vi "Check Wired Terminal.vi"(10 "Type Descriptor":T4, 11 "Terminal Type":variant) -> (3 "Terminal Status":T1)   [LabVIEW 2022 SP3, in "FlexBlocks Support.lvlib"]
uses:
  FlexBlocks Support.lvlib
  Type Descriptor.ctl
  Terminal Direction.ctl
  Value Mode.ctl
  Special Terminal.ctl
  Terminal Status.ctl
  Terminal State.ctl
  Terminal Draw Style.ctl
  <vilib>/Utility/Data Type/NI_Data Type.lvlib
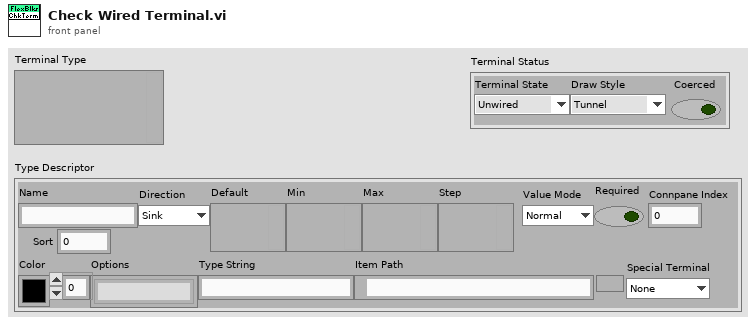
[diagram p1: front panel]
types:
  T1 = typedef "FlexBlocks Support.lvlib/Terminal Status.ctl" = cluster{"Terminal State":T2, "Draw Style":T3, "Coerced":bool}
  T2 = typedef "FlexBlocks Support.lvlib/Terminal State.ctl" = enum16{"Unwired", "BadType", "BadRef", "Channel", "Value", "Control Ref"}
  T3 = typedef "FlexBlocks Support.lvlib/Terminal Draw Style.ctl" = enum16{"Tunnel", "BadType", "BadRef", "Channel", "Value", "Control Ref"}
  T4 = typedef "FlexBlocks Support.lvlib/Type Descriptor.ctl" = cluster{"Name":string, "Direction":T5, "Default":variant, "Min":variant, "Max":variant, "Step":variant, "Value Mode":T6, "Color":u32, "Options":string[], "Type String":string, "Item Path":path, "Required":bool, "Connpane Index":i32, "Special Terminal":T7, "Sort":i32}
  T5 = typedef "FlexBlocks Support.lvlib/Terminal Direction.ctl" = enum16{"Sink", "Source"}
  T6 = typedef "FlexBlocks Support.lvlib/Value Mode.ctl" = enum16{"Normal", "Range", "Select"}
  T7 = typedef "FlexBlocks Support.lvlib/Special Terminal.ctl" = enum16{"None", "Action", "Init", "Tag", "State in", "State out", "Error"}
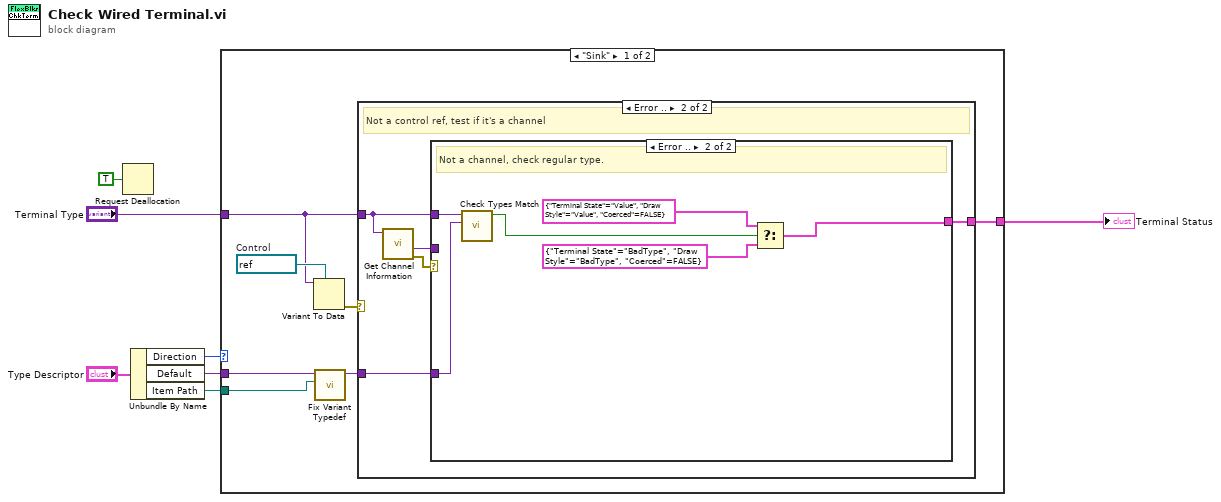
[diagram p0: block diagram]
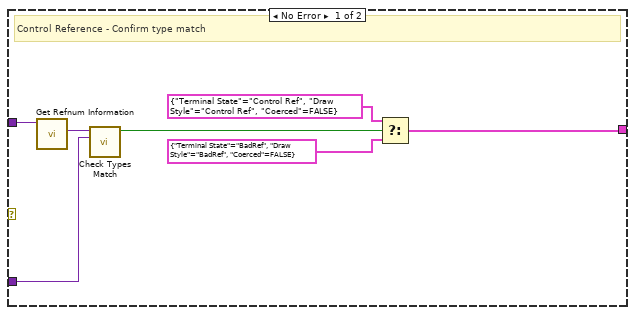
[diagram p2: hidden frame]
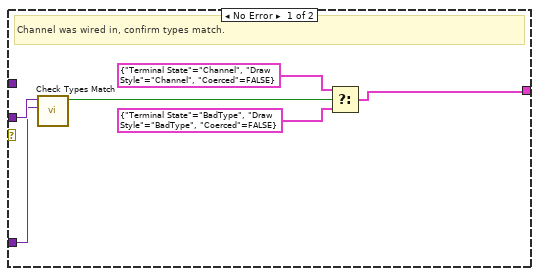
[diagram p3: hidden frame]
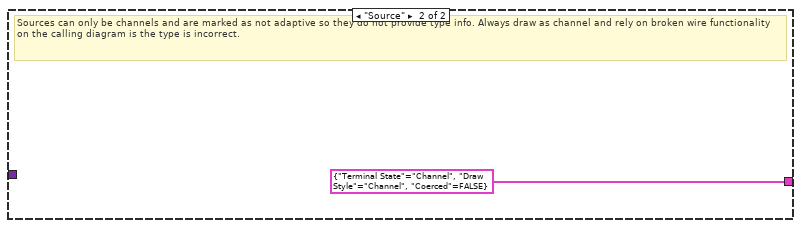
[diagram p4: hidden frame]
diagram:
  n1 = Request Deallocation(TRUE ("flag")) -> ()
  n2 = Unbundle By Name("Type Descriptor") -> ("Direction"=w1:T5, "Default"=w4:variant, "Item Path"=w3:path)
  n3 = case shown="\"Sink\"" w1 {
    tunnel: "Terminal Type" -> [w13 _]
    tunnel: w4 -> [w11 _]
    tunnel: w3 -> [w10 _]
    tunnel: [w8 T1 {"Terminal State"=enum."Channel", "Draw Style"=enum."Channel", "Coerced"=FALSE} ("Terminal Status")] -> w2
    frame "Sink" {
      w14 = refnum<vi> refnum  # Control
      n4 = Variant To Data(type=w14, Variant=w13) -> (error out=w12:errorcluster)  [unwired: 1 in, 1 out]
      n5 = call "Fix Variant Typedef.vi"("Item Path"=w10, "Default"=w11) -> ("Fixed Variant"=w9:variant)  [unwired: 9 in]
      n6 = case shown="Error .." w12 {
        tunnel: w13 -> [w21 w22]
        tunnel: w9 -> [w19 w24]
        tunnel: [w15 w23] -> w8
        frame No Error {
          # "Control Reference - Confirm type match"
          n7 = call <vilib>:"Get Refnum Information.vi"("variant"=w21) -> ("strict type"=w20:variant)  [unwired: 7 in, 3 out]
          n8 = call "Check Types Match.vi"("Type 2"=w19, "Type 1"=w20) -> ("Match?"=w18:bool)  [unwired: 9 in]
          n9 = Select(t=T1 {"Terminal State"=enum."Control Ref", "Draw Style"=enum."Control Ref", "Coerced"=FALSE} ("Terminal Status"), s=w18, f=T1 {"Terminal State"=enum."BadRef", "Draw Style"=enum."BadRef", "Coerced"=FALSE} ("Terminal Status")) -> (s? t:f=w15:T1)
        }
        frame Error {
          # "Not a control ref, test if it's a channel"
          n10 = call <vilib>:"Get Channel Information.vi"("variant"=w22) -> ("error out"=w26:errorcluster, "element type"=w25:variant)  [unwired: 6 in, 3 out]
          n11 = case shown="Error .." w26 {
            tunnel: w25 -> [w32 _]
            tunnel: w24 -> [w31 w37]
            tunnel: [w27 w33] -> w23
            tunnel: w22 -> [_ w38]
            frame No Error {
              # "Channel was wired in, confirm types match."
              n12 = call "Check Types Match.vi"("Type 2"=w31, "Type 1"=w32) -> ("Match?"=w28:bool)  [unwired: 9 in]
              n13 = Select(t=T1 {"Terminal State"=enum."Channel", "Draw Style"=enum."Channel", "Coerced"=FALSE} ("Terminal Status"), s=w28, f=T1 {"Terminal State"=enum."BadType", "Draw Style"=enum."BadType", "Coerced"=FALSE} ("Terminal Status")) -> (s? t:f=w27:T1)
            }
            frame Error {
              # "Not a channel, check regular type."
              n14 = call "Check Types Match.vi"("Type 2"=w37, "Type 1"=w38) -> ("Match?"=w34:bool)  [unwired: 9 in]
              n15 = Select(t=T1 {"Terminal State"=enum."Value", "Draw Style"=enum."Value", "Coerced"=FALSE} ("Terminal Status"), s=w34, f=T1 {"Terminal State"=enum."BadType", "Draw Style"=enum."BadType", "Coerced"=FALSE} ("Terminal Status")) -> (s? t:f=w33:T1)
            }
          }
        }
      }
    }
    frame "Source" {
      # "Sources can only be channels and are marked as not adaptive so they do not provide type info. Always draw as channel and rely on broken wire functionality on the calling diagram is the type is incorrect."
    }
  }
  "Terminal Status" <- w2
